vi "练习3.1-可变频率波形发生器.vi"() -> ()   [LabVIEW 2021]
panel:
  in  "频率":dbl
  out "Waveform Graph":dynamicdata(graph)
  in  "stop":bool
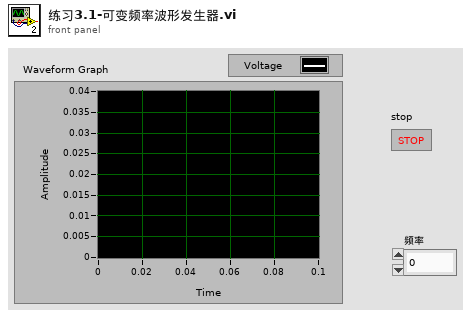
[diagram p1: front panel]
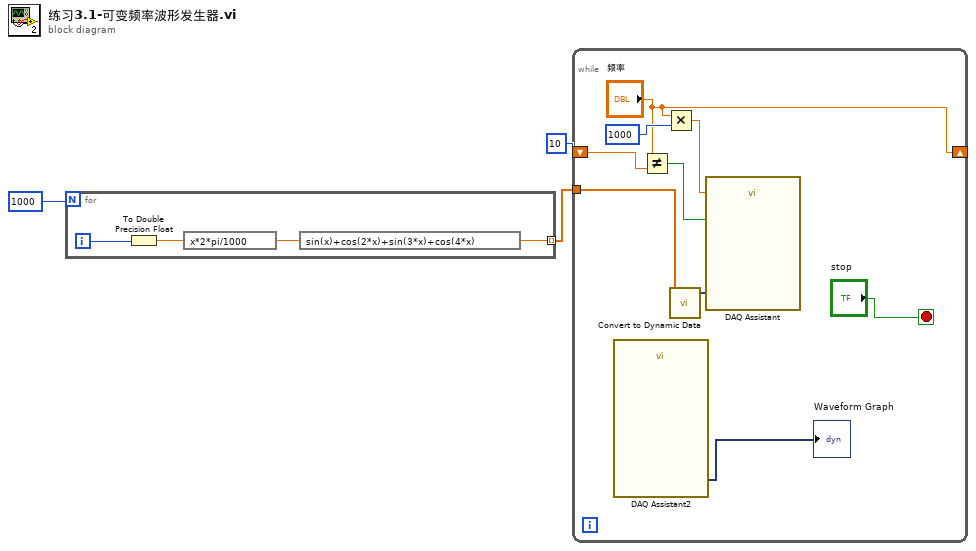
[diagram p0: block diagram]
diagram:
  n1 = for {
    N: 1000 -> [_]
    tunnel: [w4] -> w2 mode=indexing
    i -> [w7]
    n2 = To Double Precision Float(number=w7) -> (double precision float=w6:dbl)
    n3 = expression code="x*2*pi/1000"(w6) -> (w5:dbl)
    n4 = expression code="sin(x)+cos(2*x)+sin(3*x)+cos(4*x)"(w5) -> (w4:dbl)
  }
  n5 = while {
    tunnel: w2 -> [w15]
    shift-right: ["频率"] -> _
    shift-left: 10 -> [w12]
    stop <- "stop" stop-if-true
    n6 = call "DAQ Assistant2"() -> ("data"=→"Waveform Graph":dynamicdata)  [unwired: 17 in, 2 out]
    n7 = Not Equal?(x="频率", y=w12) -> (x != y?=w11:bool)
    n8 = Multiply(x="频率", y=1000) -> (x*y=w9:dbl)
    n9 = call "Convert to Dynamic Data"("Array"=w15) -> ("Dynamic Data Type"=w14:dynamicdata)  [unwired: 3 in]
    n10 = call "DAQ Assistant"("data"=w14, "rate"=w9, "stop (F)"=w11) -> ()  [unwired: 14 in, 3 out]
  }
